vi "set_store_path.vi"(8 "error in (no error)":errorcluster, 10 "error file store path":path, 11 "ErrorController in":refnum<class "ErrorController.lvclass">) -> (0 "error out":errorcluster, 3 "ErrorController out":refnum<class "ErrorController.lvclass">)   [LabVIEW 2010, in "ErrorController.lvclass"]
uses:
  ErrorController.lvclass
  ErrorController.lvclass/ErrorController.ctl
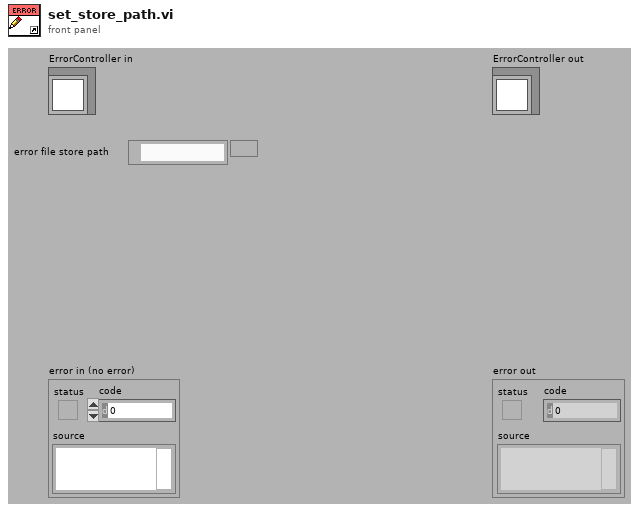
[diagram p1: front panel]
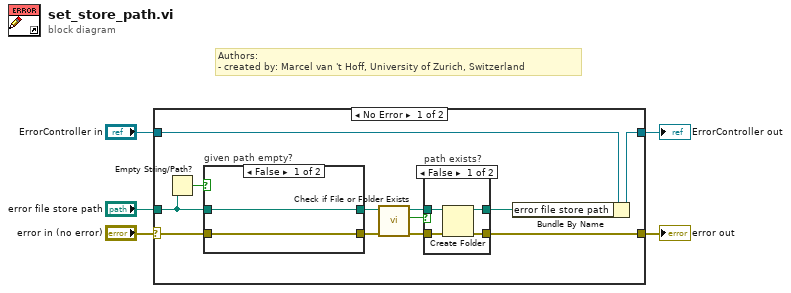
[diagram p0: block diagram]
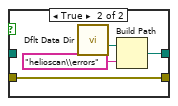
[diagram p2: hidden frame]
diagram:
  # "Authors: \n- created by: Marcel van 't Hoff, University of Zurich, Switzerland"
  n1 = case shown="No Error" "error in (no error)" {
    selector: "error in (no error)" -> [w9 w31]
    tunnel: [w14 w31] -> w4
    tunnel: [w16 w30] -> w2
    tunnel: "ErrorController in" -> [w17 w30]
    tunnel: "error file store path" -> [w6 _]
    frame No Error {
      n2 = Empty String/Path?(string/path=w6) -> (empty?=w7:bool)
      n3 = case "given path empty?" shown="False" w7 {
        tunnel: [w18 w21] -> w13
        tunnel: w9 -> [w19 w20]
        tunnel: [w19 w20] -> w8
        tunnel: w6 -> [w18 _]
        frame False {
        }
        frame True {
          n4 = call <vilib>:"Dflt Data Dir.vi"() -> ("App:Default Data Directory"=w23:path)
          n5 = Build Path(base path=w23, name or relative path="helioscan\\errors") -> (appended path=w21:path)
        }
      }
      n6 = call <vilib>:"Check if File or Folder Exists.vi"("error in (no error)"=w8, "path"=w13) -> ("error out"=w10:errorcluster, "file or folder exists?"=w12:bool, "dup path"=w11:path)  [unwired: 7 in]
      n7 = case "path exists?" shown="False" w12 {
        tunnel: w11 -> [w27 w29]
        tunnel: [w25 w29] -> w15
        tunnel: w10 -> [w26 w28]
        tunnel: [w24 w28] -> w14
        frame False {
          n8 = Create Folder(path (use dialog)=w27, error in=w26) -> (created path=w25:path, error out=w24:errorcluster)  [unwired: 1 in, 1 out]
        }
        frame True {
        }
      }
      n9 = Bundle By Name(cluster=w17, "error file store path"=w15) -> (w16:refnum<class "ErrorController.lvclass">)
    }
    frame Error {
    }
  }
  "error out" <- w4
  "ErrorController out" <- w2
